vi "Compute Possible Connections.vi"(8 "error in":errorcluster, 11 "slsc switch custom device in":T2 format="%.0x") -> (0 "error out":errorcluster, 2 "possible connections":T1[](array[typedef]), 3 "slsc switch custom device out":T2 format="%.0x")   [LabVIEW 2020, in "SLSC Switch Scripting.lvlib"]
uses:
  SLSC Switch Scripting.lvlib
  <vilib>/NI VeriStand/Custom Device API/Custom Device Item Ref.ctl
  Routing and Faulting/Routing and Faulting Hardware API/Types/Possible Connections for Endpoint.ctl
  <vilib>/SLSC_Switch/Initialize with Topology (Simulate).vi
  <vilib>/SLSC_Switch/SLSC Switch.lvlib
  Routing and Faulting/Routing and Faulting Hardware API/Routing and Faulting Hardware API.lvlib
  <vilib>/NI VeriStand/Custom Device API/Custom Device API.lvlib
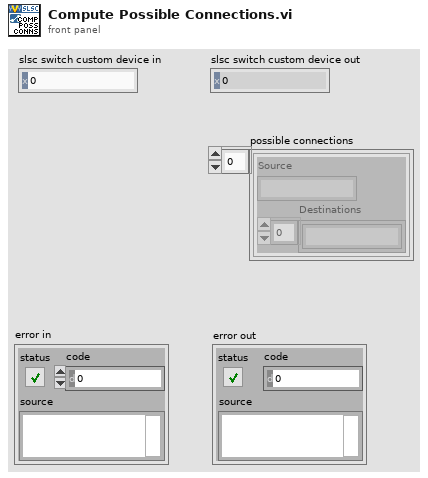
[diagram p1: front panel]
types:
  T1 = typedef "Routing and Faulting Hardware API.lvlib/Possible Connections for Endpoint.ctl" = cluster{"Source":string, "Destinations":string[]}
  T2 = typedef "Custom Device API.lvlib/Custom Device Item Ref.ctl" = u64
  T3 = typedef "nislscslSession.ctl" = refnum<k20>
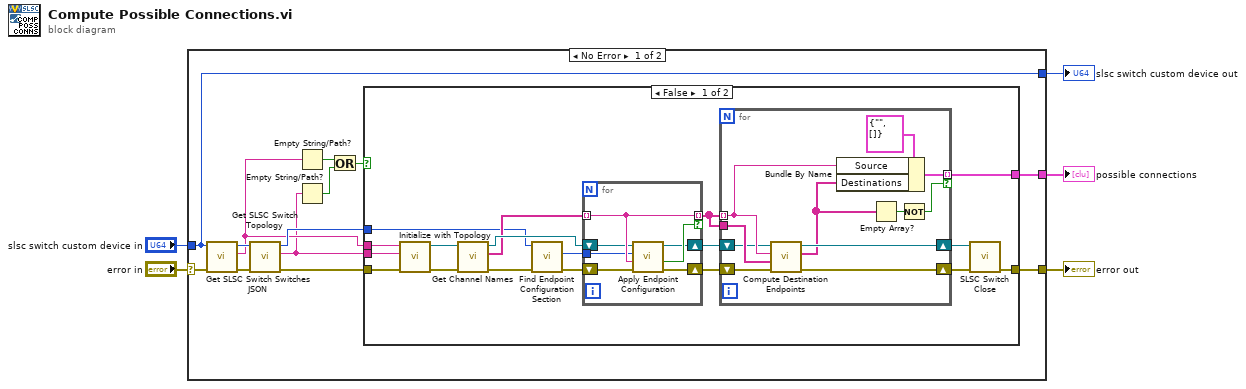
[diagram p0: block diagram]
diagram:
  n1 = case shown="No Error" "error in" {
    selector: "error in" -> [w14 w57]
    tunnel: [w18 w57] -> w5
    tunnel: "slsc switch custom device in" -> [w8 w56]
    tunnel: [w8 w56] -> w3
    tunnel: [w12 _] -> w1
    frame No Error {
      n2 = call "Get SLSC Switch Switches JSON.vi"("error in"=w14, "slsc switch custom device in"=w8) -> ("error out"=w17:errorcluster, "switches json"=w11:string, "slsc switch custom device out"=w16:T2)  [unwired: 7 in]
      n3 = call "Get SLSC Switch Topology.vi"("error in"=w17, "slsc switch custom device in"=w16) -> ("error out"=w13:errorcluster, "topology"=w10:string, "slsc switch custom device out"=w15:T2)  [unwired: 7 in]
      n4 = Empty String/Path?(string/path=w11) -> (empty?=w6:bool)
      n5 = Empty String/Path?(string/path=w10) -> (empty?=w7:bool)
      n6 = Or(x=w6, y=w7) -> (x .or. y?=w9:bool)
      n7 = case shown="False" w9 {
        tunnel: [w27 w55] -> w18
        tunnel: w11 -> [w26 _]
        tunnel: w10 -> [w25 _]
        tunnel: w15 -> [w20 _]
        tunnel: w13 -> [w24 w55]
        tunnel: [w23 _] -> w12
        frame False {
          n8 = call-poly <vilib>:"Initialize with Topology.vi"("error in (no error)"=w24, "topology"=w25, "switches json"=w26) -> ("error out"=w32:errorcluster, "session out"=w35:T3)  [unwired: 7 in]
          n9 = call <vilib>:"Get Channel Names.vi"("error in (no error)"=w32, "session in"=w35) -> ("error out"=w22:errorcluster, "channel names"=w33:string[], "session out"=w34:T3)  [unwired: 7 in]
          n10 = call "Find Endpoint Configuration Section.vi"("error in"=w22, "slsc switch custom device in"=w20) -> ("error out"=w21:errorcluster, "endpoint configuration"=w19:T2)  [unwired: 7 in, 1 out]
          n11 = for {
            tunnel: [w40] -> w36 mode=indexing if=w43
            tunnel: w33 -> [w40] mode=indexing
            tunnel: w19 -> [w38]
            shift-right: [w41] -> w31
            shift-left: w21 -> [w42]
            shift-right: [w37] -> w30
            shift-left: w34 -> [w39]
            n12 = call "Apply Endpoint Configuration.vi"("error in"=w42, "endpoint"=w40, "endpoint configuration in"=w38, "slsc switch session in"=w39) -> ("error out"=w41:errorcluster, "endpoint addressable?"=w43:bool, "slsc switch session out"=w37:T3)  [unwired: 4 in, 1 out]
          }
          n13 = for {
            tunnel: w36 -> [w49] mode=indexing
            tunnel: w36 -> [w54]
            shift-right: [w52] -> w29
            shift-left: w31 -> [w53]
            shift-right: [w51] -> w28
            shift-left: w30 -> [w44]
            tunnel: [w46] -> w23 mode=indexing if=w45
            n14 = call "Compute Destination Endpoints.vi"("error in"=w53, "endpoints"=w54, "source endpoint"=w49, "slsc switch session in"=w44) -> ("error out"=w52:errorcluster, "possible destinations"=w47:string[], "slsc switch session out"=w51:T3)  [unwired: 5 in]
            n15 = Bundle By Name(cluster=T1 {"Source"="", "Destinations"=[]} ("Possible Connections for Endpoint"), "Source"=w49, "Destinations"=w47) -> (w46:T1)
            n16 = Empty Array?(array=w47) -> (empty?=w48:bool)
            n17 = Not(x=w48) -> (.not. x?=w45:bool)
          }
          n18 = call "SLSC Switch Close.vi"("error in"=w29, "slsc switch session"=w28) -> ("error out"=w27:errorcluster)  [unwired: 9 in]
        }
        frame True {
        }
      }
    }
    frame Error {
    }
  }
  "error out" <- w5
  "slsc switch custom device out" <- w3
  "possible connections" <- w1
